vi "Destroy M1M3 Support Events.vi"(8 "error in (no error)":errorcluster, 11 "M1M3 Support Events in":refnum<class "M1M3 Support Events.lvclass">) -> (0 "error out":errorcluster, 3 "M1M3 Support Events out":refnum<class "M1M3 Support Events.lvclass">)   [LabVIEW 2016, in "M1M3 Support Events.lvclass"]
uses:
  M1M3 Support Events.lvclass
  M1M3 Support Events.lvclass/M1M3 Support Events.ctl
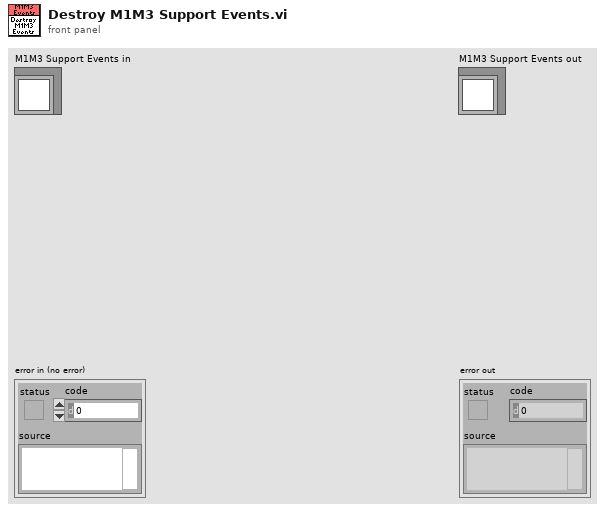
[diagram p1: front panel]
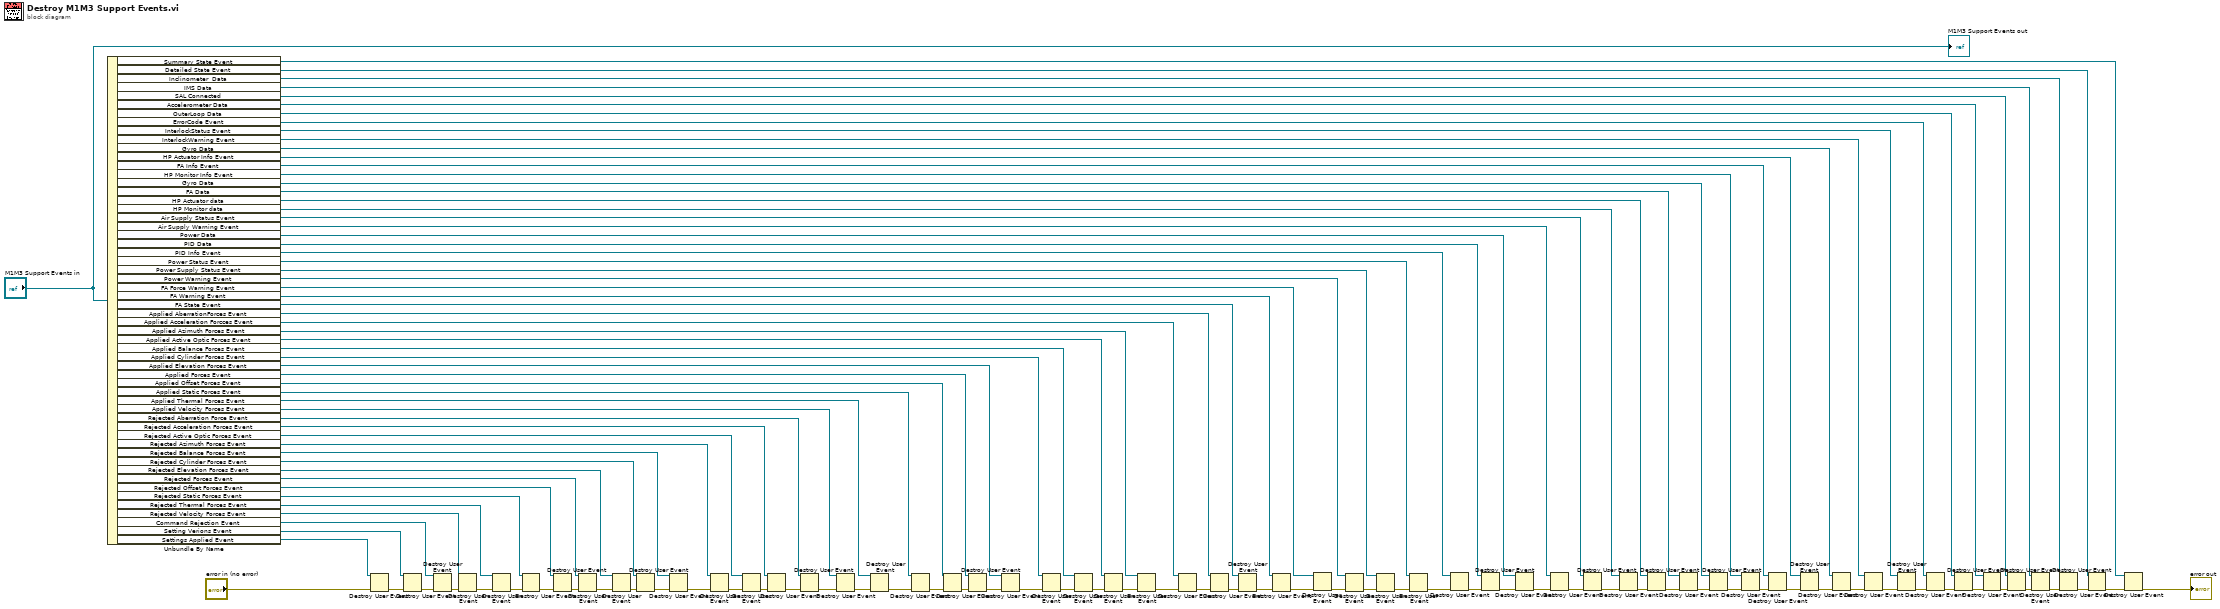
[diagram p0: block diagram]
diagram:
  n1 = Unbundle By Name("M1M3 Support Events in") -> ("Summary State Event"=w62:refnum<user-event>, "Detailed State Event"=w107:refnum<user-event>, "Inclinometer  Data"=w108:refnum<user-event>, "IMS Data"=w109:refnum<user-event>, "SAL Connected"=w114:refnum<user-event>, "Accelerometer Data"=w103:refnum<user-event>, "OuterLoop Data"=w104:refnum<user-event>, "ErrorCode Event"=w105:refnum<user-event>, "InterlockStatus Event"=w106:refnum<user-event>, "InterlockWarning Event"=w97:refnum<user-event>, "Gyro Data"=w93:refnum<user-event>, "HP Actuator Info Event"=w92:refnum<user-event>, "FA Info Event"=w91:refnum<user-event>, "HP Monitor Info Event"=w89:refnum<user-event>, "Gyro Data"=w87:refnum<user-event>, "FA Data"=w84:refnum<user-event>, "HP Actuator data"=w83:refnum<user-event>, "HP Monitor data"=w82:refnum<user-event>, "Air Supply Status Event"=w77:refnum<user-event>, "Air Supply Warning Event"=w78:refnum<user-event>, "Power Data"=w74:refnum<user-event>, "PID Data"=w73:refnum<user-event>, "PID Info Event"=w71:refnum<user-event>, "Power Status Event"=w67:refnum<user-event>, "Power Supply Status Event"=w66:refnum<user-event>, "Power Warning Event"=w65:refnum<user-event>, "FA Force Warning Event"=w58:refnum<user-event>, "FA Warning Event"=w57:refnum<user-event>, "FA State Event"=w56:refnum<user-event>, "Applied AberrationForces Event"=w43:refnum<user-event>, "Applied Acceleration Forcces Event"=w42:refnum<user-event>, "Applied Azimuth Forces Event"=w41:refnum<user-event>, "Applied Active Optic Forces Event"=w40:refnum<user-event>, "Applied Balance Forces Event"=w39:refnum<user-event>, "Applied Cylinder Forces Event"=w38:refnum<user-event>, "Applied Elevation Forces Event"=w37:refnum<user-event>, "Applied Forces Event"=w36:refnum<user-event>, "Applied Offset Forces Event"=w35:refnum<user-event>, "Applied Static Forces Event"=w34:refnum<user-event>, "Applied Thermal Forces Event"=w33:refnum<user-event>, "Applied Velocity Forces Event"=w32:refnum<user-event>, "Rejected Aberration Force Event"=w19:refnum<user-event>, "Rejected Acceleration Forces Event"=w18:refnum<user-event>, "Rejected Active Optic Forces Event"=w17:refnum<user-event>, "Rejected Azimuth Forces Event"=w16:refnum<user-event>, "Rejected Balance Forces Event"=w15:refnum<user-event>, "Rejected Cylinder Forces Event"=w14:refnum<user-event>, "Rejected Elevation Forces Event"=w13:refnum<user-event>, "Rejected Forces Event"=w12:refnum<user-event>, "Rejected Offset Forces Event"=w11:refnum<user-event>, "Rejected Static Forces Event"=w10:refnum<user-event>, "Rejected Thermal Forces Event"=w9:refnum<user-event>, "Rejected Velocity Forces Event"=w8:refnum<user-event>, "Command Rejection Event"=w3:refnum<user-event>, "Setting Verions Event"=w2:refnum<user-event>, "Settings Applied Event"=w1:refnum<user-event>)
  n2 = Destroy User Event(user event=w1, error in="error in (no error)") -> (error out=w6:errorcluster)
  n3 = Destroy User Event(user event=w2, error in=w6) -> (error out=w7:errorcluster)
  n4 = Destroy User Event(user event=w3, error in=w7) -> (error out=w5:errorcluster)
  n5 = Destroy User Event(user event=w8, error in=w5) -> (error out=w24:errorcluster)
  n6 = Destroy User Event(user event=w9, error in=w24) -> (error out=w23:errorcluster)
  n7 = Destroy User Event(user event=w10, error in=w23) -> (error out=w25:errorcluster)
  n8 = Destroy User Event(user event=w11, error in=w25) -> (error out=w22:errorcluster)
  n9 = Destroy User Event(user event=w12, error in=w22) -> (error out=w26:errorcluster)
  n10 = Destroy User Event(user event=w13, error in=w26) -> (error out=w20:errorcluster)
  n11 = Destroy User Event(user event=w14, error in=w20) -> (error out=w29:errorcluster)
  n12 = Destroy User Event(user event=w15, error in=w29) -> (error out=w30:errorcluster)
  n13 = Destroy User Event(user event=w16, error in=w30) -> (error out=w28:errorcluster)
  n14 = Destroy User Event(user event=w17, error in=w28) -> (error out=w31:errorcluster)
  n15 = Destroy User Event(user event=w18, error in=w31) -> (error out=w27:errorcluster)
  n16 = Destroy User Event(user event=w19, error in=w27) -> (error out=w21:errorcluster)
  n17 = Destroy User Event(user event=w32, error in=w21) -> (error out=w48:errorcluster)
  n18 = Destroy User Event(user event=w33, error in=w48) -> (error out=w47:errorcluster)
  n19 = Destroy User Event(user event=w34, error in=w47) -> (error out=w49:errorcluster)
  n20 = Destroy User Event(user event=w35, error in=w49) -> (error out=w44:errorcluster)
  n21 = Destroy User Event(user event=w36, error in=w44) -> (error out=w51:errorcluster)
  n22 = Destroy User Event(user event=w37, error in=w51) -> (error out=w52:errorcluster)
  n23 = Destroy User Event(user event=w38, error in=w52) -> (error out=w50:errorcluster)
  n24 = Destroy User Event(user event=w39, error in=w50) -> (error out=w45:errorcluster)
  n25 = Destroy User Event(user event=w40, error in=w45) -> (error out=w54:errorcluster)
  n26 = Destroy User Event(user event=w41, error in=w54) -> (error out=w53:errorcluster)
  n27 = Destroy User Event(user event=w42, error in=w53) -> (error out=w55:errorcluster)
  n28 = Destroy User Event(user event=w43, error in=w55) -> (error out=w46:errorcluster)
  n29 = Destroy User Event(user event=w56, error in=w46) -> (error out=w60:errorcluster)
  n30 = Destroy User Event(user event=w57, error in=w60) -> (error out=w61:errorcluster)
  n31 = Destroy User Event(user event=w58, error in=w61) -> (error out=w59:errorcluster)
  n32 = Destroy User Event(user event=w65, error in=w59) -> (error out=w70:errorcluster)
  n33 = Destroy User Event(user event=w66, error in=w70) -> (error out=w69:errorcluster)
  n34 = Destroy User Event(user event=w67, error in=w69) -> (error out=w68:errorcluster)
  n35 = Destroy User Event(user event=w71, error in=w68) -> (error out=w72:errorcluster)
  n36 = Destroy User Event(user event=w73, error in=w72) -> (error out=w75:errorcluster)
  n37 = Destroy User Event(user event=w74, error in=w75) -> (error out=w76:errorcluster)
  n38 = Destroy User Event(user event=w78, error in=w76) -> (error out=w80:errorcluster)
  n39 = Destroy User Event(user event=w77, error in=w80) -> (error out=w79:errorcluster)
  n40 = Destroy User Event(user event=w82, error in=w79) -> (error out=w81:errorcluster)
  n41 = Destroy User Event(user event=w83, error in=w81) -> (error out=w85:errorcluster)
  n42 = Destroy User Event(user event=w84, error in=w85) -> (error out=w86:errorcluster)
  n43 = Destroy User Event(user event=w87, error in=w86) -> (error out=w88:errorcluster)
  n44 = Destroy User Event(user event=w89, error in=w88) -> (error out=w90:errorcluster)
  n45 = Destroy User Event(user event=w91, error in=w90) -> (error out=w95:errorcluster)
  n46 = Destroy User Event(user event=w92, error in=w95) -> (error out=w96:errorcluster)
  n47 = Destroy User Event(user event=w93, error in=w96) -> (error out=w94:errorcluster)
  n48 = Destroy User Event(user event=w97, error in=w94) -> (error out=w98:errorcluster)
  n49 = Destroy User Event(user event=w106, error in=w98) -> (error out=w99:errorcluster)
  n50 = Destroy User Event(user event=w105, error in=w99) -> (error out=w100:errorcluster)
  n51 = Destroy User Event(user event=w104, error in=w100) -> (error out=w101:errorcluster)
  n52 = Destroy User Event(user event=w103, error in=w101) -> (error out=w102:errorcluster)
  n53 = Destroy User Event(user event=w114, error in=w102) -> (error out=w112:errorcluster)
  n54 = Destroy User Event(user event=w109, error in=w112) -> (error out=w111:errorcluster)
  n55 = Destroy User Event(user event=w108, error in=w111) -> (error out=w110:errorcluster)
  n56 = Destroy User Event(user event=w107, error in=w110) -> (error out=w64:errorcluster)
  n57 = Destroy User Event(user event=w62, error in=w64) -> (error out=→"error out":errorcluster)
  "M1M3 Support Events out" <- "M1M3 Support Events in"
